vi "Format LLP Data for Display.vi"(9 "packet index offset":u64, 11 "tagged packets":T1[](array[typedef])) -> (3 "display data":string[][](array[string]))   [LabVIEW 2023, in "GettingStarted_Common_148X_Host.lvlib"]
uses:
  GettingStarted_Common_148X_Host.lvlib
  <instrlib>/FlexRIO/CSI-2/v2/Host/Types/Host Tagged LLP Packet.ctl
  <instrlib>/FlexRIO/CSI-2/v2/Host/Types/Host LLP Packet Tag.ctl
  <instrlib>/FlexRIO/CSI-2/v2/Host/Types/Host LLP Packet Timestamp.ctl
  <instrlib>/FlexRIO/CSI-2/v2/FPGA/Types/Timestamp ID.ctl
  <instrlib>/FlexRIO/CSI-2/v2/Host/Types/Host LLP Packet Size.ctl
  <instrlib>/FlexRIO/CSI-2/v2/Host/Types/Host LLP Packet.ctl
  <instrlib>/FlexRIO/CSI-2/v2/FPGA/Types/LLP Packet Header.ctl
  <instrlib>/FlexRIO/CSI-2/v2/FPGA/Types/LLP Packet Footer.ctl
  <instrlib>/FlexRIO/CSI-2/v2/Common/Types/LLP Data Type.ctl
  <instrlib>/FlexRIO/CSI-2/v2/Common/NI CSI-2 API Common v2.lvlib
  <instrlib>/FlexRIO/CSI-2/v2/FPGA/NI CSI-2 API FPGA v2.lvlib
  <instrlib>/FlexRIO/CSI-2/v2/Host/NI CSI-2 API Host v2.lvlib
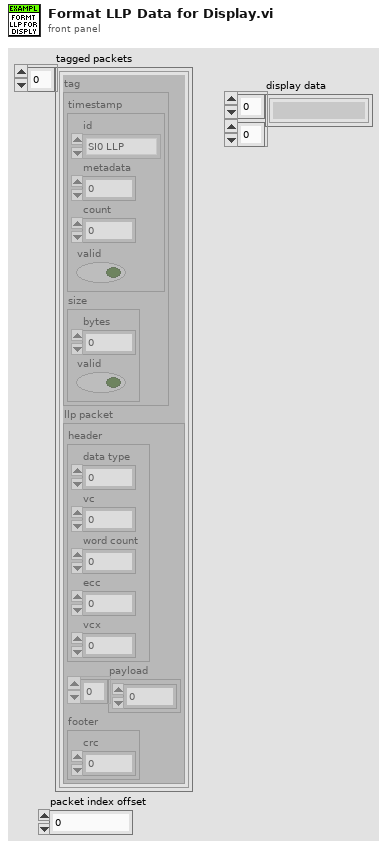
[diagram p1: front panel]
types:
  T1 = typedef "NI CSI-2 API Host v2.lvlib/Host Tagged LLP Packet.ctl" = cluster{"tag":T2, "llp packet":T6}
  T2 = typedef "NI CSI-2 API Host v2.lvlib/Host LLP Packet Tag.ctl" = cluster{"timestamp":T3, "size":T5}
  T3 = typedef "NI CSI-2 API Host v2.lvlib/Host LLP Packet Timestamp.ctl" = cluster{"valid":bool, "count":u64, "id":T4, "metadata":u8}
  T4 = typedef "NI CSI-2 API FPGA v2.lvlib/Timestamp ID.ctl" = enum8{"SI0 LLP", "SI1 LLP", "SI2 LLP", "SI3 LLP", "SI4 LLP", "SI5 LLP", "SI6 LLP", "SI7 LLP", "SO0 LLP", "SO1 LLP", "SO2 LLP", "SO3 LLP", "SO4 LLP", "SO5 LLP", "SO6 LLP", "SO7 LLP", "Ser0 GPIO Bank", "Ser1 GPIO Bank", "Ser2 GPIO Bank", "Ser3 GPIO Bank", "Ser4 GPIO Bank", "Ser5 GPIO Bank", "Ser6 GPIO Bank", "Ser7 GPIO Bank", "Des0 GPIO Bank", "Des1 GPIO Bank", "Des2 GPIO Bank", "Des3 GPIO Bank", "Des4 GPIO Bank", "Des5 GPIO Bank", "Des6 GPIO Bank", "Des7 GPIO Bank", "User0", "User1", "User2", "User3", "User4", "User5", "User6", "User7", "User8", "User9", "User10", "User11", "User12", "User13", "User14", "User15", "User16", "User17", "User18", "User19", "User20", "User21", "User22", "User23", "User24", "User25", "User26", "User27", "User28", "User29", "User30", "User31"}
  T5 = typedef "NI CSI-2 API Host v2.lvlib/Host LLP Packet Size.ctl" = cluster{"bytes":u32, "valid":bool}
  T6 = typedef "NI CSI-2 API Host v2.lvlib/Host LLP Packet.ctl" = cluster{"header":T7, "payload":u8[], "footer":T8}
  T7 = typedef "NI CSI-2 API FPGA v2.lvlib/LLP Packet Header.ctl" = cluster{"word count":u16, "ecc":fxp<+,6,6>, "vcx":fxp<+,2,2>, "data type":fxp<+,6,6>, "vc":fxp<+,2,2>}
  T8 = typedef "NI CSI-2 API FPGA v2.lvlib/LLP Packet Footer.ctl" = cluster{"crc":u16}
  T9 = typedef "NI CSI-2 API Common v2.lvlib/LLP Data Type.ctl" = enum8{"Frame Start", "Frame End", "Line Start", "Line End", "End of Transmission", "Reserved 0", "Reserved 1", "Reserved 2", "Generic Short Packet 1", "Generic Short Packet 2", "Generic Short Packet 3", "Generic Short Packet 4", "Generic Short Packet 5", "Generic Short Packet 6", "Generic Short Packet 7", "Generic Short Packet 8", "Null", "Blanking Data", "Embedded 8-bit non Image Data", "Generic Long Packet 1", "Generic Long Packet 2", "Generic Long Packet 3", "Generic Long Packet 4", "Reserved 3", "YUV420 8-bit", "YUV420 10-bit", "Legacy YUV420 8-bit", "Reserved 4", "YUV420 8-bit Chroma Shifted", "YUV420 10-bit Chroma Shifted", "YUV422 8-bit", "YUV422 10-bit", "RGB444", "RGB555", "RGB565", "RGB666", "RGB888", "Reserved 5", "Reserved 6", "RAW 24", "RAW 6", "RAW 7", "RAW 8", "RAW 10", "RAW 12", "RAW 14", "RAW 16", "RAW 20", "User Defined 8-bit Data 1", "User Defined 8-bit Data 2", "User Defined 8-bit Data 3", "User Defined 8-bit Data 4", "User Defined 8-bit Data 5", "User Defined 8-bit Data 6", "User Defined 8-bit Data 7", "User Defined 8-bit Data 8", "USL Command", "Reserved 7", "Reserved 8", "Reserved 9", "Reserved 10", "Reserved 11", "Reserved 12", "LRTE EPD Spacer"}
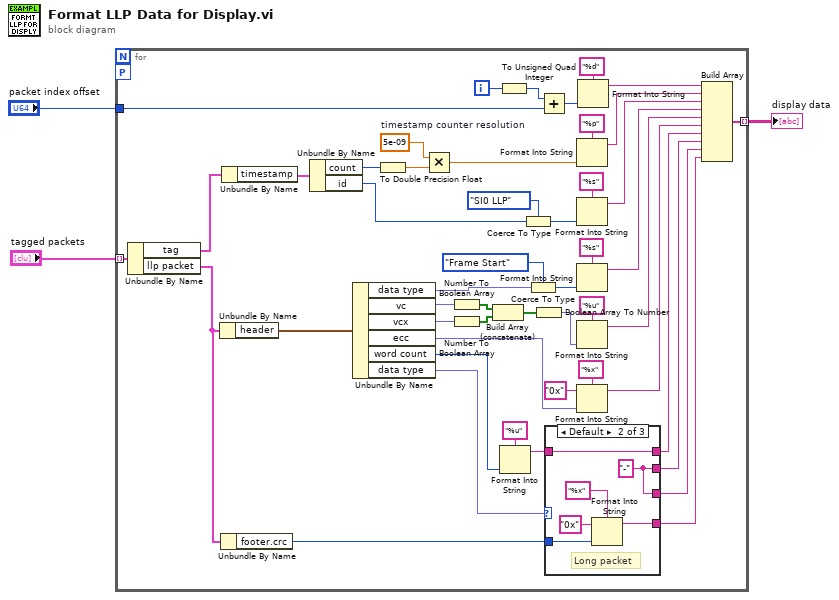
[diagram p0: block diagram]
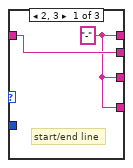
[diagram p2: hidden frame]
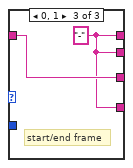
[diagram p3: hidden frame]
diagram:
  n1 = for {
    tunnel: [w50] -> w3 mode=indexing
    workers-P: _ -> [_]
    tunnel: "packet index offset" -> [w11]
    tunnel: "tagged packets" -> [w7] mode=indexing
    i -> [w9]
    w17 = 5e-09  # timestamp counter resolution
    n2 = Unbundle By Name(w7) -> ("tag"=w6:T2, "llp packet"=w5:T6)
    n3 = Unbundle By Name(w5) -> ("header"=w52:T7)
    n4 = Unbundle By Name(w5) -> ("footer.crc"=w20:u16)
    n5 = Unbundle By Name(w6) -> ("timestamp"=w4:T3)
    n6 = Unbundle By Name(w4) -> ("count"=w16:u64, "id"=w42:T4)
    n7 = Unbundle By Name(w52) -> ("data type"=w49:fxp<+,6,6>, "vc"=w36:fxp<+,2,2>, "vcx"=w35:fxp<+,2,2>, "ecc"=w30:fxp<+,6,6>, "word count"=w27:u16, "data type"=w25:fxp<+,6,6>)
    n8 = To Double Precision Float(number=w16) -> (double precision float=w15:dbl)
    n9 = Multiply(x=w17, y=w15) -> (x*y=w18:dbl)
    n10 = Number To Boolean Array(number=w36) -> (Boolean array=w38:bool[])
    n11 = Number To Boolean Array(number=w35) -> (Boolean array=w37:bool[])
    n12 = Build Array (concatenate)(w38, w37) -> (w39:bool[])
    n13 = To Unsigned Quad Integer(1:w9) -> (0:w8:u64)
    n14 = Format Into String(format string="%u", w27) -> (resulting string=w24:string)  [unwired: 2 in, 1 out]
    n15 = Coerce To Type(0:w42, 1:Timestamp_ID."SI0 LLP" ("id")) -> (2:w44:T4)
    n16 = Coerce To Type(0:w49, 1:LLP_Data_Type."Frame Start" ("Enum")) -> (2:w47:T9)
    n17 = Boolean Array To Number(Boolean array=w39) -> (number=w33:fxp<+,4,4>)
    n18 = Add(x=w8, y=w11) -> (x+y=w10:u64)
    n19 = case shown="Default" w25 {
      tunnel: w24 -> [w54 w60 w62]
      tunnel: [w53 w60 w61] -> w23
      tunnel: [w54 w59 w61] -> w22
      tunnel: [w53 w59 w62] -> w21
      tunnel: w20 -> [_ w56 _]
      tunnel: [w53 w55 w61] -> w19
      frame 2, 3 {
        w53 = "-"
        # "start/end line"
      }
      frame Default {
        w59 = "-" ("format string")
        # "Long packet"
        n20 = Format Into String(format string="%x", initial string="0x", w56) -> (resulting string=w55:string)  [unwired: 1 in, 1 out]
      }
      frame 0, 1 {
        w61 = "-"
        # "start/end frame"
      }
    }
    n21 = Format Into String(format string="%p", w18) -> (resulting string=w51:string)  [unwired: 2 in, 1 out]
    n22 = Format Into String(format string="%s", w44) -> (resulting string=w40:string)  [unwired: 2 in, 1 out]
    n23 = Format Into String(format string="%s", w47) -> (resulting string=w41:string)  [unwired: 2 in, 1 out]
    n24 = Format Into String(format string="%u", w33) -> (resulting string=w32:string)  [unwired: 2 in, 1 out]
    n25 = Format Into String(format string="%x", initial string="0x", w30) -> (resulting string=w29:string)  [unwired: 1 in, 1 out]
    n26 = Format Into String(format string="%d", w10) -> (resulting string=w12:string)  [unwired: 2 in, 1 out]
    n27 = Build Array(w12, w51, w40, w41, w32, w29, w23, w22, w21, w19) -> (w50:string[])
  }
  "display data" <- w3
